vi "picture2image.vi"(8 "error in (no error)":errorcluster, 11 "data_loader in":refnum<class "data_loader.lvclass">) -> (0 "error out":errorcluster, 3 "data_loader out":refnum<class "data_loader.lvclass">)   [LabVIEW 2017, in "data_loader.lvclass"]
uses:
  data_loader.lvclass
  data_loader.lvclass/data_loader.ctl
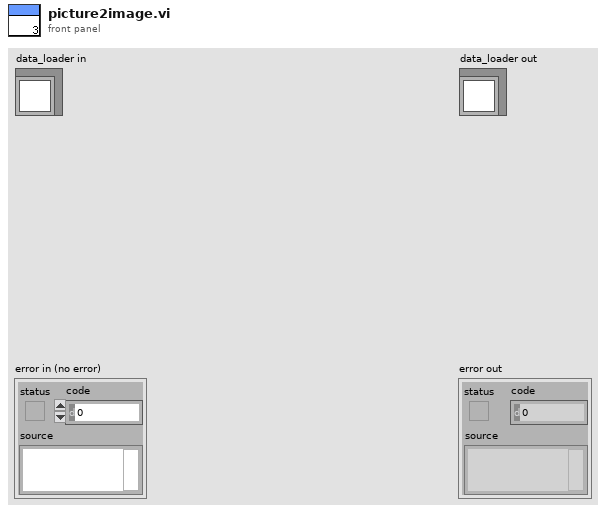
[diagram p1: front panel]
types:
  T1 = typedef "Image Type" = u32
  T2 = typedef "imagedata.ctl" = cluster{"image type":i32, "image depth":i32, "image":u8[], "mask":u8[], "colors":u32[], "Rectangle":cluster{"left":i16, "top":i16, "right":i16, "bottom":i16}}
  T3 = typedef "IMAQ Image.ctl" = refnum<image>
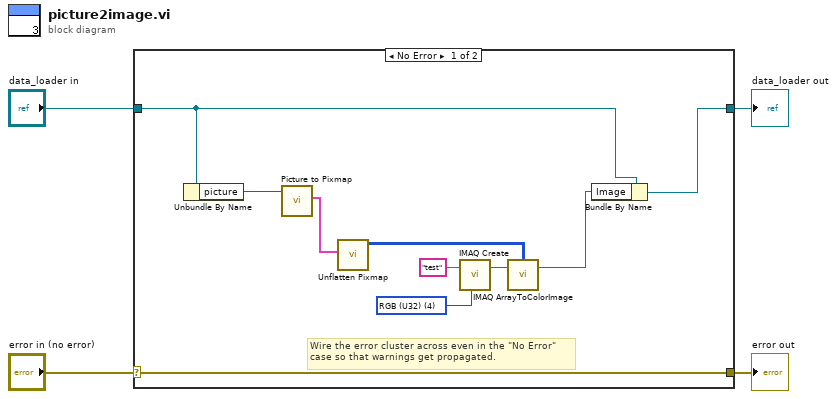
[diagram p0: block diagram]
diagram:
  n1 = case shown="No Error" "error in (no error)" {
    selector: "error in (no error)" -> [w14 w16]
    tunnel: [w14 w16] -> w3
    tunnel: [w5 w15] -> w1
    tunnel: "data_loader in" -> [w6 w15]
    frame No Error {
      w11 = T1 4 items=["Grayscale (U8)", "Grayscale (I16)", "Grayscale (SGL)", "Complex (CSG)", "RGB (U32)", "HSL (U32)", "RGB (U64)", "Grayscale (U16)"] ("Image Type")
      # "Wire the error cluster across even in the \"No Error\"\ncase so that warnings get propagated."
      n2 = Unbundle By Name(w6) -> ("picture"=w8:picture)
      n3 = call <vilib>:"Picture to Pixmap.vi"("picture"=w8) -> ("image data"=w9:T2)  [unwired: 9 in, 1 out]
      n4 = call <vilib>:"Unflatten Pixmap.vi"("image data"=w9) -> ("24-bit pixmap"=w10:u32[][])  [unwired: 4 in, 6 out]
      n5 = call "IMAQ Create"("Image Name"="test", "Image Type"=w11) -> ("New Image"=w13:T3)  [unwired: 3 in, 1 out]
      n6 = call "IMAQ ArrayToColorImage"("Image Pixels (U32)"=w10, "Image"=w13) -> ("Image Out"=w7:T3)  [unwired: 3 in, 1 out]
      n7 = Bundle By Name(cluster=w6, "Image"=w7) -> (w5:refnum<class "data_loader.lvclass">)
    }
    frame Error {
    }
  }
  "error out" <- w3
  "data_loader out" <- w1
